vi "ROI entry-Line entry handler.vi"(8 "error in (no error)":errorcluster, 10 "Coordinates":i32[](array[numeric]), 11 "Tool":i32) -> (0 "error out":errorcluster, 1 "Do not generate line ROI":bool, 3 "Array":T1[](array[typedef]) {"Zoom" min=1.0 max=10.0 step=0.10000000149011612})   [LabVIEW 2013]
uses:
  Typedefs/ROI spec.ctl
  Typedefs/ROI ID Enum.ctl
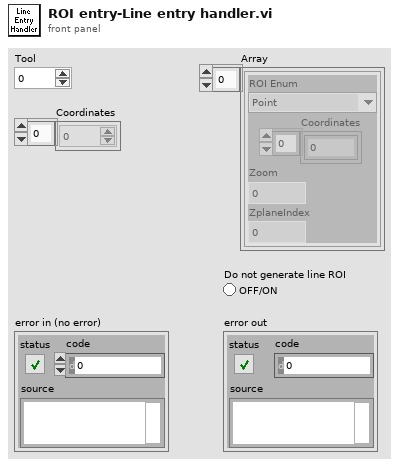
[diagram p1: front panel]
types:
  T1 = typedef "ROI spec.ctl" = cluster{"Coordinates":i32[], "Zoom":dbl, "ROI Enum":T2, "ZplaneIndex":i32}
  T2 = typedef "ROI ID Enum.ctl" = enum16{"Point", "MiniScan", "Comp. MiniScan", "Rectangle", "Comp. volume", "Arb. plane point"}
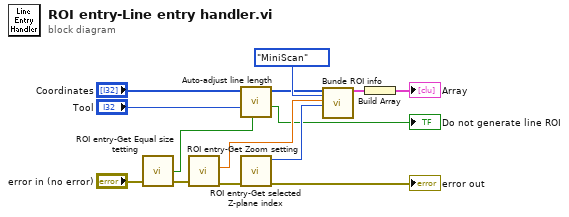
[diagram p0: block diagram]
diagram:
  n1 = call "ROI entry-Get Equal size tetting.vi"("error in (no error)"="error in (no error)") -> ("error out"=w13:errorcluster, "Equal size setting's value"=w8:bool)  [unwired: 3 in]
  n2 = call "ROI entry-Get Zoom setting.vi"("error in (no error)"=w13) -> ("error out"=w14:errorcluster, "Zoom Value"=w7:dbl)  [unwired: 8 in, 1 out]
  n3 = call "Auto-adjust line length.vi"("Equal size"=w8, "Current ROI Tool"="Tool", "New Coordinates"="Coordinates") -> ("Do not generate ROI"=→"Do not generate line ROI":bool, "Output coordinates"=w5:i32[])  [unwired: 6 in, 1 out]
  n4 = call "ROI entry-Get selected Z-plane index.vi"("error in (no error)"=w14) -> ("error out"=→"error out":errorcluster, "Z-plane selector (index)"=w11:i32)  [unwired: 9 in]
  n5 = call "Bunde ROI info.vi"("ROI Coordinates"=w5, "ROI Enum"=ROI_ID_Enum."MiniScan", "Zoom"=w7, "ZplaneIndex"=w11) -> ("ROI Info"=w3:T1)  [unwired: 15 in]
  n6 = Build Array(w3) -> (→"Array":T1[])
